vi "MakeLiquid.vi"(9 "level":dbl, 10 "tank":T1, 11 "room_temperature":dbl) -> (3 "liquid":T2)   [LabVIEW 2020]
uses:
  Liquid.ctl
  TankResolution.ctl
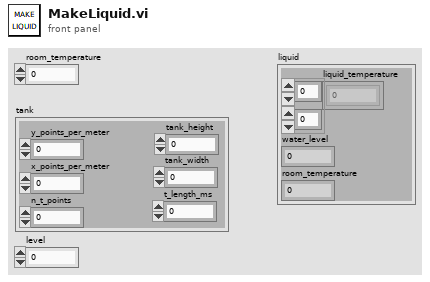
[diagram p1: front panel]
types:
  T1 = typedef "TankResolution.ctl" = cluster{"y_points_per_meter":i32, "x_points_per_meter":i32, "n_t_points":i32, "tank_height":dbl, "tank_width":dbl, "t_length_ms":u32}
  T2 = typedef "Liquid.ctl" = cluster{"liquid_temperature":dbl[][], "water_level":dbl, "room_temperature":dbl}
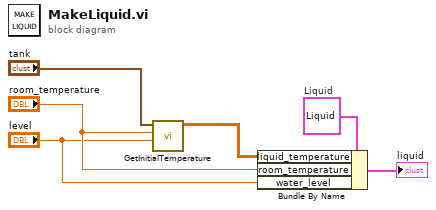
[diagram p0: block diagram]
diagram:
  w6 = T2 {"liquid_temperature"=array75x50[3750 elements], "water_level"=1.4948979591836733, "room_temperature"=298.15}  # Liquid
  n1 = call "GetInitialTemperature.vi"("level"="level", "room_temperature"="room_temperature", "tank_resolution"="tank") -> ("initial_temperature"=w5:dbl[][])  [unwired: 8 in]
  n2 = Bundle By Name(cluster=w6, "liquid_temperature"=w5, "room_temperature"="room_temperature", "water_level"="level") -> (→"liquid":T2)
